vi "Exemple_Preprocessing_PowerTransformer.vi"() -> ()   [LabVIEW 2020]
uses:
  Objet/6 - Datasets Transformation/6.3 - Processing Data/PowerTransformer/PowerTransformer.lvclass
panel:
  in  "y":string[][](array[string])
  in  "X":string[][](array[string])=[["1", "2"], ["3", "2"], ["4", "5"]]
  out "Data":T1
  out "error out":errorcluster
  in  "error in":errorcluster caption="entrée d'erreur"
  in  "PowerTransformer":T2={"method"="yeo-johnson", "standardize"=TRUE, "copy"=TRUE}
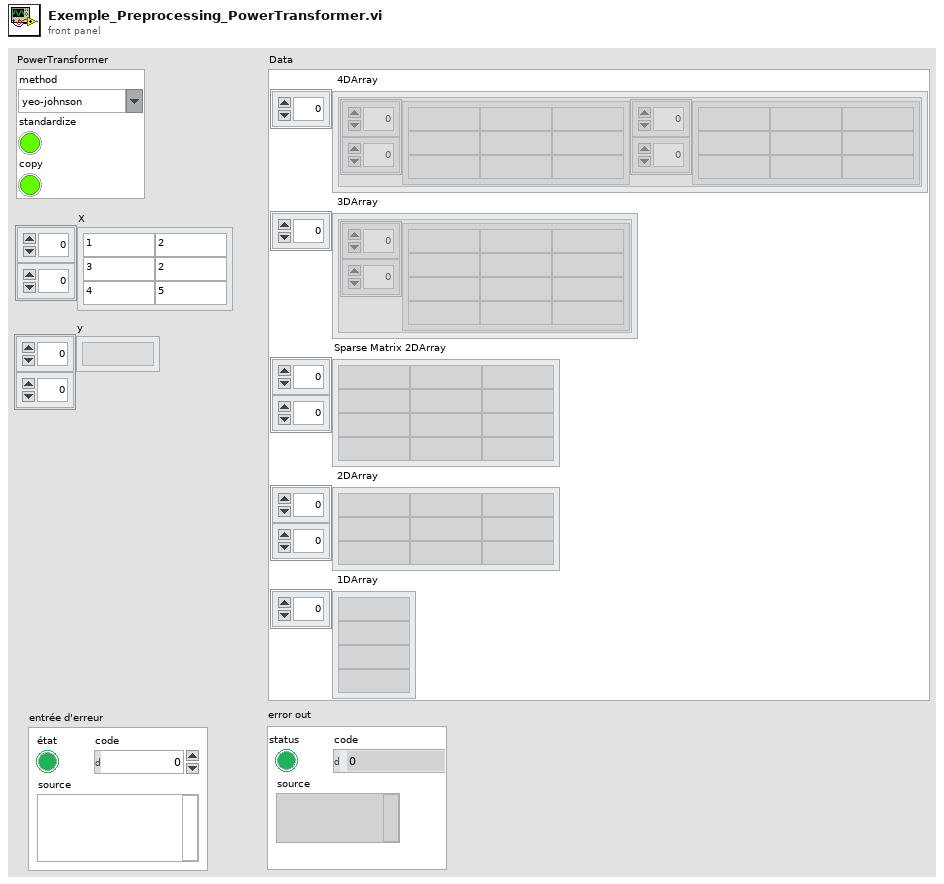
[diagram p1: front panel]
types:
  T1 = cluster{" 4DArray":cluster{"1":string[][], "2":string[][]}[], " 3DArray":cluster{"Tableau":string[][]}[], "Sparse Matrix 2DArray":string[][], " 2DArray":string[][], " 1DArray":string[]}
  T2 = cluster{"method":string, "standardize":bool, "copy":bool}
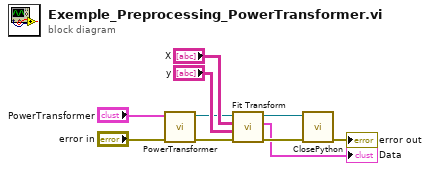
[diagram p0: block diagram]
diagram:
  n1 = call "PowerTransformer.vi"("error in (no error)"="error in", "PowerTransformer"="PowerTransformer") -> ("error out"=w9:errorcluster, "PowerTransformer.lvclass"=w6:refnum<class "PowerTransformer.lvclass">)  [unwired: 8 in]
  n2 = call-dynamic "Fit Transform.vi"("error in (no error)"=w9, "y"="y", "X"="X", "PowerTransformer.lvclass"=w6) -> ("error out"=w4:errorcluster, "Data"=→"Data":T1, "PowerTransformer.lvclass"=w5:refnum<class "PowerTransformer.lvclass">)  [unwired: 5 in]
  n3 = call-dynamic "ClosePython.vi"("error in (no error)"=w4, "Scikit-learn en entrée"=w5) -> ("error out"=→"error out":errorcluster)  [unwired: 8 in, 1 out]
